vi "REV Robotics Analog Pressur Sensor.vi"(6 "Vcc (V)":dbl=5.0, 7 "Median Filter Rank":i32=25, 8 "error in (no error)":errorcluster, 11 "Vout (V)":dbl) -> (0 "error out":errorcluster, 3 "Pressure (PSI)":dbl)   [LabVIEW 2018]
uses:
  <vilib>/Utility/error.llb/Error Cluster From Error Code.vi
  <vilib>/ErrorRing/Error Ring.xnode
  <vilib>/ptbypt/NI_PtbyPt.lvlib
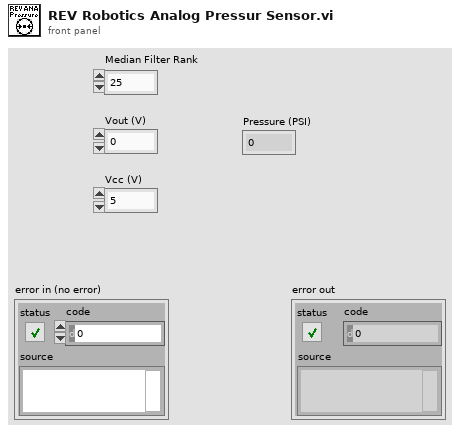
[diagram p1: front panel]
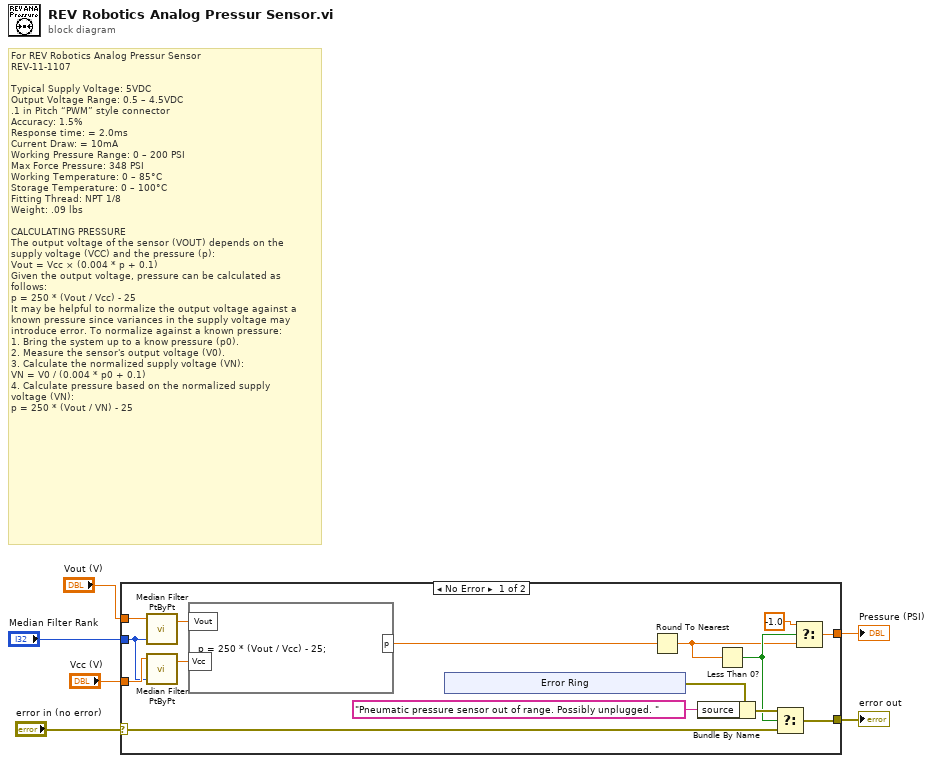
[diagram p0: block diagram]
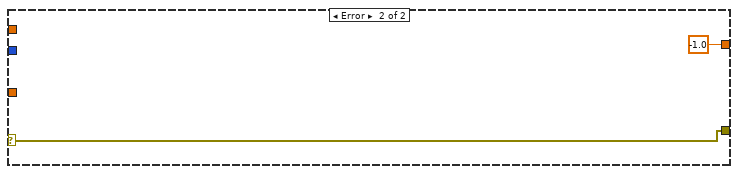
[diagram p2: hidden frame]
diagram:
  # "For REV Robotics Analog Pressur Sensor\nREV-11-1107\n\nTypical Supply Voltage: 5VDC\nOutput Voltage Range: 0.5 – 4.5VDC\n.1 in Pitch “PWM” style connector\nAccuracy: 1.5%\nResponse time: = 2.0ms\nCurrent Draw: = 10mA\nWorking Pressure Range: 0 – 200 PSI\nMax Force Pressure: 348 PSI\nWorking Temperature: 0 – 85°C\nStorage Temperature: 0 – 100°C\nFitting Thread: NPT 1/8\nWeight: .09 lbs\n\nCALCULATING PRESSURE\nThe output voltage of the sensor (VOUT) depends on the\nsupply voltage (VCC) and the pressure (p):\nVout = Vcc × (0.004 * p + 0.1)\nGiven the output voltage, pressure can be calculated as\nfollows:\np = 250 * (Vout / Vcc) - 25\nIt may be helpful to normalize the output voltage against a\nknown pressure since variances in the supply voltage may\nintroduce error. To normalize against a known pressure:\n1. Bring the system up to a know pressure (p0).\n2. Measure the sensor's output voltage (V0).\n3. Calculate the normalized supply voltage (VN):\nVN = V0 / (0.004 * p0 + 0.1)\n4. Calculate pressure based on the normalized supply\nvoltage (VN):\np = 250 * (Vout / VN) - 25"
  n1 = case shown="No Error" "error in (no error)" {
    selector: "error in (no error)" -> [w15 w27]
    tunnel: [w8 -1.0] -> w6
    tunnel: "Vout (V)" -> [w20 _]
    tunnel: "Vcc (V)" -> [w18 _]
    tunnel: "Median Filter Rank" -> [w16 _]
    tunnel: [w14 w27] -> w1
    frame No Error {
      n2 = call <vilib>:"Median Filter PtByPt.vi"("rank"=w16, "x"=w20) -> ("Filtered x"=w19:dbl)  [unwired: 2 in, 1 out]
      n3 = call <vilib>:"Median Filter PtByPt.vi"("rank"=w16, "x"=w18) -> ("Filtered x"=w17:dbl)  [unwired: 2 in, 1 out]
      n4 = formula code="p = 250 * (Vout / Vcc) - 25;"("Vout"=w19, "Vcc"=w17) -> ("p"=w21:dbl)
      n5 = xnode "Error Ring"() -> ("error out"=w13:errorcluster)
      n6 = Round To Nearest(number=w21) -> (nearest integer value=w9:dbl)
      n7 = Bundle By Name(cluster=w13, "source"="Pneumatic pressure sensor out of range. Possibly unplugged. ") -> (w11:errorcluster)
      n8 = Less Than 0?(x=w9) -> (x < 0?=w10:bool)
      n9 = Select(t=w11, s=w10, f=w15) -> (s? t:f=w14:errorcluster)
      n10 = Select(t=-1.0, s=w10, f=w9) -> (s? t:f=w8:dbl)
    }
    frame Error {
    }
  }
  "Pressure (PSI)" <- w6
  "error out" <- w1
